vi "data_waypoint_ref.vi"() -> ()   [LabVIEW 2019] (continued)
"Y"=530169.107673044}, {"X"=175301.515584441, "Y"=530169.1522306317}, {"X"=175301.5505684368, "Y"=530169.1965216612}, {"X"=175301.58586430468, "Y"=530169.2408384063}, {"X"=175301.621437572, "Y"=530169.2849046132}, {"X"=175301.65624651004, "Y"=530169.3287078214}, {"X"=175301.69067446323, "Y"=530169.3715787638}, {"X"=175301.72433513994, "Y"=530169.4131889531}, {"X"=175301.7572057744, "Y"=530169.4545273413}, {"X"=175301.7897156011, "Y"=530169.4957669071}, {"X"=175301.82262842666, "Y"=530169.5363948606}, {"X"=175301.85541520052, "Y"=530169.5775315022}, {"X"=175301.88877971005, "Y"=530169.6193356836}, {"X"=175301.92198627733, "Y"=530169.6622479695}, {"X"=175301.9549979493, "Y"=530169.7066524813}, {"X"=175301.98874946675, "Y"=530169.7514277223}, {"X"=175302.02408231725, "Y"=530169.7962715428}, {"X"=175302.05988879167, "Y"=530169.84162117}, {"X"=175302.09521931363, "Y"=530169.886875645}, {"X"=175302.12915909418, "Y"=530169.9324128029}, {"X"=175302.16313239714, "Y"=530169.9770042623}, {"X"=175302.19741865405, "Y"=530170.0198878336}, {"X"=175302.23161996814, "Y"=530170.0622022983}, {"X"=175302.2647214002, "Y"=530170.1043091388}, {"X"=175302.29732747353, "Y"=530170.1466471837}, {"X"=175302.32942471874, "Y"=530170.1900533064}, {"X"=175302.36214685687, "Y"=530170.2339004164}, {"X"=175302.39546431036, "Y"=530170.2777679664}, {"X"=175302.42970125427, "Y"=530170.3213508952}, {"X"=175302.46371953157, "Y"=530170.3649755353}, {"X"=175302.4970483943, "Y"=530170.409108309}, {"X"=175302.53014454423, "Y"=530170.452725684}, {"X"=175302.56359763598, "Y"=530170.4957338027}, {"X"=175302.59699459223, "Y"=530170.5389285439}, {"X"=175302.63076028306, "Y"=530170.5819079936}, {"X"=175302.6641188947, "Y"=530170.625916373}, {"X"=175302.6977430426, "Y"=530170.6704567027}, {"X"=175302.7314268824, "Y"=530170.7154141635}, {"X"=175302.76559054904, "Y"=530170.7605799701}, {"X"=175302.80000400502, "Y"=530170.8048449432}, {"X"=175302.83450216462, "Y"=530170.8486979064}, {"X"=175302.868423361, "Y"=530170.8930431358}, {"X"=175302.9020594507, "Y"=530170.9368298354}, {"X"=175302.93501567593, "Y"=530170.9804587241}, {"X"=175302.96820232505, "Y"=530171.0238283353}, {"X"=175303.0014239085, "Y"=530171.0667294834}, {"X"=175303.03441731303, "Y"=530171.1100519415}, {"X"=175303.06691230068, "Y"=530171.153469102}, {"X"=175303.09917383848, "Y"=530171.1964219182}, {"X"=175303.13118923537, "Y"=530171.2397117508}, {"X"=175303.1637000194, "Y"=530171.2824795955}, {"X"=175303.19595648517, "Y"=530171.3261138815}, {"X"=175303.22875163666, "Y"=530171.3703914051}, {"X"=175303.26162110508, "Y"=530171.4149395159}, {"X"=175303.2943639709, "Y"=530171.4604080732}, {"X"=175303.3270933593, "Y"=530171.5061119605}, {"X"=175303.36078521397, "Y"=530171.5507863855}, {"X"=175303.39476642053, "Y"=530171.5950592977}, {"X"=175303.42826067653, "Y"=530171.6391105651}, {"X"=175303.46060070378, "Y"=530171.683447147}, {"X"=175303.4932010295, "Y"=530171.7277418941}, {"X"=175303.5264554045, "Y"=530171.7715508118}, {"X"=175303.56027406864, "Y"=530171.815673263}, {"X"=175303.59372100336, "Y"=530171.8604982444}, {"X"=175303.62725594908, "Y"=530171.9051320691}, {"X"=175303.66013932397, "Y"=530171.9501906737}, {"X"=175303.69312924595, "Y"=530171.9947339906}, {"X"=175303.72571887134, "Y"=530172.0390054631}, {"X"=175303.75856571438, "Y"=530172.0833916041}, {"X"=175303.7914979888, "Y"=530172.1276121215}, {"X"=175303.82426099747, "Y"=530172.1724058269}, {"X"=175303.85658823774, "Y"=530172.2175126894}, {"X"=175303.8893403862, "Y"=530172.2622276273}, {"X"=175303.9219982045, "Y"=530172.3070960032}, {"X"=175303.95487855875, "Y"=530172.3514321018}, {"X"=175303.98756941865, "Y"=530172.395190523}, {"X"=175304.0198873744, "Y"=530172.4383540505}, {"X"=175304.05146210626, "Y"=530172.4803022576}, {"X"=175304.08243248635, "Y"=530172.5218682386}, {"X"=175304.11302771606, "Y"=530172.5638781629}, {"X"=175304.14440576072, "Y"=530172.6058125234}, {"X"=175304.17647083785, "Y"=530172.6485317448}, {"X"=175304.2092485257, "Y"=530172.6916983553}, {"X"=175304.2421544904, "Y"=530172.7351098659}, {"X"=175304.27474581596, "Y"=530172.7793591394}, {"X"=175304.30713692037, "Y"=530172.8241972291}, {"X"=175304.33966600779, "Y"=530172.8692668731}, {"X"=175304.3725380399, "Y"=530172.9146862191}, {"X"=175304.40615073708, "Y"=530172.9595551069}, {"X"=175304.43922888403, "Y"=530173.0045820643}, {"X"=175304.47193721798, "Y"=530173.0500607167}, {"X"=175304.50408048517, "Y"=530173.095561017}, {"X"=175304.53664703757, "Y"=530173.1407204481}, {"X"=175304.57019344828, "Y"=530173.1850401526}, {"X"=175304.60417604624, "Y"=530173.229188761}, {"X"=175304.63733822326, "Y"=530173.274475177}, {"X"=175304.67012666404, "Y"=530173.3200845581}, {"X"=175304.70293440312, "Y"=530173.3656295104}, {"X"=175304.73601901694, "Y"=530173.4107485677}, {"X"=175304.7688052838, "Y"=530173.4550216836}, {"X"=175304.80180875398, "Y"=530173.4984595454}, {"X"=175304.83439683876, "Y"=530173.5410129662}, {"X"=175304.86641084577, "Y"=530173.5832384543}, {"X"=175304.89706473134, "Y"=530173.6259163404}, {"X"=175304.92851563115, "Y"=530173.6676274072}, {"X"=175304.96001501603, "Y"=530173.7089609802}, {"X"=175304.9911972434, "Y"=530173.7511778257}, {"X"=175305.0218017102, "Y"=530173.7939191228}, {"X"=175305.0528701443, "Y"=530173.8368965593}, {"X"=175305.0845467455, "Y"=530173.8803494384}, {"X"=175305.11676661787, "Y"=530173.9241980441}, {"X"=175305.1485606208, "Y"=530173.9687116023}, {"X"=175305.1810053819, "Y"=530174.0134252321}, {"X"=175305.21403351048, "Y"=530174.0580150564}, {"X"=175305.24728412752, "Y"=530174.1035575917}, {"X"=175305.28061614945, "Y"=530174.1499689076}, {"X"=175305.31471056672, "Y"=530174.1962902915}, {"X"=175305.3486507356, "Y"=530174.243170392}, {"X"=175305.3823800229, "Y"=530174.2900289173}, {"X"=175305.4154933949, "Y"=530174.3367893738}, {"X"=175305.4486278848, "Y"=530174.3826019497}, {"X"=175305.48151879795, "Y"=530174.4275195878}, {"X"=175305.5138967311, "Y"=530174.4724010066}, {"X"=175305.54595081756, "Y"=530174.517701799}, {"X"=175305.57926572644, "Y"=530174.562519407}, {"X"=175305.61313334163, "Y"=530174.6076283868}, {"X"=175305.64742550213, "Y"=530174.6531223445}, {"X"=175305.68094282097, "Y"=530174.6995930464}, {"X"=175305.7142195681, "Y"=530174.7464862061}, {"X"=175305.74732664338, "Y"=530174.7932144965}, {"X"=175305.78057287785, "Y"=530174.8402742251}, {"X"=175305.8133739154, "Y"=530174.8877536852}, {"X"=175305.84608374408, "Y"=530174.9352422942}, {"X"=175305.8802467283, "Y"=530174.9825878779}, {"X"=175305.91585264518, "Y"=530175.02962732}, {"X"=175305.95117603574, "Y"=530175.0772802396}, {"X"=175305.98675250847, "Y"=530175.1248480605}, {"X"=175306.0226269634, "Y"=530175.1719366532}, {"X"=175306.05766248834, "Y"=530175.219295199}, {"X"=175306.09146300732, "Y"=530175.2665819227}, {"X"=175306.1256061778, "Y"=530175.3138176922}, {"X"=175306.15987830423, "Y"=530175.3612284362}, {"X"=175306.19375731278, "Y"=530175.4089977182}, {"X"=175306.2272617157, "Y"=530175.4570955143}, {"X"=175306.26149442443, "Y"=530175.5043554353}, {"X"=175306.29601557076, "Y"=530175.5512049651}, {"X"=175306.33110052024, "Y"=530175.5979052205}, {"X"=175306.3664420601, "Y"=530175.6445070498}, {"X"=175306.40137430347, "Y"=530175.6922876495}, {"X"=175306.43611313298, "Y"=530175.7405627077}, {"X"=175306.47135692826, "Y"=530175.7888606924}, {"X"=175306.50683563814, "Y"=530175.836619701}, {"X"=175306.5427093849, "Y"=530175.8837704501}, {"X"=175306.57804036967, "Y"=530175.9312979346}, {"X"=175306.61314321528, "Y"=530175.9786596134}, {"X"=175306.64723720393, "Y"=530176.0260398111}, {"X"=175306.68197792507, "Y"=530176.0728576195}, {"X"=175306.71729545467, "Y"=530176.1191287831}, {"X"=175306.75288187485, "Y"=530176.1655689615}, {"X"=175306.78805515857, "Y"=530176.2121868278}, {"X"=175306.82317604765, "Y"=530176.2593597791}, {"X"=175306.85816065417, "Y"=530176.3068771907}, {"X"=175306.89302999235, "Y"=530176.3543549852}, {"X"=175306.92829042548, "Y"=530176.4019892259}, {"X"=175306.96434128538, "Y"=530176.4494269079}, {"X"=175307.0002629, "Y"=530176.4974909314}, {"X"=175307.03651319438, "Y"=530176.5461732863}, {"X"=175307.07280654478, "Y"=530176.5944370972}, {"X"=175307.10929617652, "Y"=530176.6425793526}, {"X"=175307.1459389947, "Y"=530176.6904026284}, {"X"=175307.1830941412, "Y"=530176.738340926}, {"X"=175307.2198662148, "Y"=530176.7870406077}, {"X"=175307.25608431565, "Y"=530176.836519937}, {"X"=175307.2923623031, "Y"=530176.8870823126}, {"X"=175307.32952882035, "Y"=530176.9370727075}, {"X"=175307.36630468437, "Y"=530176.9870564856}, {"X"=175307.40306440124, "Y"=530177.0369715019}, {"X"=175307.43982546963, "Y"=530177.0867444496}, {"X"=175307.47700678377, "Y"=530177.1363463515}, {"X"=175307.51413816065, "Y"=530177.1855366402}, {"X"=175307.55166098283, "Y"=530177.2347013578}, {"X"=175307.58907466935, "Y"=530177.2841050166}, {"X"=175307.62627763985, "Y"=530177.3341430286}, {"X"=175307.66311196302, "Y"=530177.3850267321}, {"X"=175307.7005225817, "Y"=530177.4357899772}, {"X"=175307.73824461747, "Y"=530177.486425782}, {"X"=175307.77605915256, "Y"=530177.5362899586}, {"X"=175307.81286147056, "Y"=530177.5865344778}, {"X"=175307.84951953805, "Y"=530177.6365241562}, {"X"=175307.88651088442, "Y"=530177.6859901074}, {"X"=175307.92401568915, "Y"=530177.7353546531}, {"X"=175307.9616221725, "Y"=530177.7846556385}, {"X"=175307.99953877402, "Y"=530177.8345883267}, {"X"=175308.03749193915, "Y"=530177.884904919}, {"X"=175308.07523145544, "Y"=530177.9354618721}, {"X"=175308.11299889255, "Y"=530177.9858755714}, {"X"=175308.15146935455, "Y"=530178.0352905402}, {"X"=175308.1892898605, "Y"=530178.0844787983}, {"X"=175308.2265397046, "Y"=530178.1335943816}, {"X"=175308.26328121778, "Y"=530178.1833474154}, {"X"=175308.30082930517, "Y"=530178.2326729915}, {"X"=175308.3391933072, "Y"=530178.2817331203}, {"X"=175308.37776592822, "Y"=530178.3309480151}, {"X"=175308.41586902775, "Y"=530178.3798457655}, {"X"=175308.45360439137, "Y"=530178.4289987606}, {"X"=175308.49054393347, "Y"=530178.4786213585}, {"X"=175308.52805617274, "Y"=530178.5275064252}, {"X"=175308.56581533956, "Y"=530178.5760211812}, {"X"=175308.60384613005, "Y"=530178.6241300373}, {"X"=175308.6412520306, "Y"=530178.6727002201}, {"X"=175308.67826697233, "Y"=530178.7214602334}, {"X"=175308.71486306612, "Y"=530178.7711648659}, {"X"=175308.75246034496, "Y"=530178.8215513228}, {"X"=175308.7912765256, "Y"=530178.872557922}, {"X"=175308.83084101314, "Y"=530178.9247021361}, {"X"=175308.8709113982, "Y"=530178.9771833654}, {"X"=175308.9109508622, "Y"=530179.0296935422}, {"X"=175308.95094127575, "Y"=530179.0814902235}, {"X"=175308.99123117467, "Y"=530179.1321184501}, {"X"=175309.03012990014, "Y"=530179.1819827599}, {"X"=175309.0674750189, "Y"=530179.2309682134}, {"X"=175309.1034754659, "Y"=530179.2796402158}, {"X"=175309.13934451604, "Y"=530179.327610065}, {"X"=175309.1753644265, "Y"=530179.3756738087}, {"X"=175309.21217135477, "Y"=530179.4232857344}, {"X"=175309.24893715564, "Y"=530179.4707690383}, {"X"=175309.28518585657, "Y"=530179.5189197841}, {"X"=175309.32090653412, "Y"=530179.5670399042}, {"X"=175309.35713197305, "Y"=530179.6151130308}, {"X"=175309.3934266228, "Y"=530179.6635266797}, {"X"=175309.42987620586, "Y"=530179.712513667}, {"X"=175309.46639058788, "Y"=530179.7624460628}, {"X"=175309.50371548356, "Y"=530179.8120852838}, {"X"=175309.5409782049, "Y"=530179.8619666371}, {"X"=175309.5787927472, "Y"=530179.9121404743}, {"X"=175309.61645778242, "Y"=530179.9635788811}, {"X"=175309.65459812188, "Y"=530180.0163932223}, {"X"=175309.69325909083, "Y"=530180.0694357668}, {"X"=175309.7317165625, "Y"=530180.122557711}, {"X"=175309.76908308847, "Y"=530180.1751967588}, {"X"=175309.80636802042, "Y"=530180.2269015467}, {"X"=175309.84373904276, "Y"=530180.2774640337}, {"X"=175309.88096197287, "Y"=530180.3267706002}, {"X"=175309.91734318458, "Y"=530180.3757034084}, {"X"=175309.9532567708, "Y"=530180.4237596989}, {"X"=175309.98798831712, "Y"=530180.472282293}, {"X"=175310.02238339974, "Y"=530180.5208502738}, {"X"=175310.0573020126, "Y"=530180.5694289177}, {"X"=175310.09330661935, "Y"=530180.6183128951}, {"X"=175310.12955154193, "Y"=530180.6672871724}, {"X"=175310.1658978246, "Y"=530180.7169914382}, {"X"=175310.20254698073, "Y"=530180.7669722736}, {"X"=175310.23967130386, "Y"=530180.817684213}, {"X"=175310.2773086728, "Y"=530180.8690550049}, {"X"=175310.3148211599, "Y"=530180.9201309427}, {"X"=175310.3511979726, "Y"=530180.9723744758}, {"X"=175310.38740139623, "Y"=530181.0252955357}, {"X"=175310.42416107788, "Y"=530181.0797110443}, {"X"=175310.4624049127, "Y"=530181.1348802013}, {"X"=175310.50164816767, "Y"=530181.1901351993}, {"X"=175310.54203527907, "Y"=530181.244894042}, {"X"=175310.58194975206, "Y"=530181.2991792613}, {"X"=175310.62001042886, "Y"=530181.3529172424}, {"X"=175310.65622358862, "Y"=530181.4049370685}, {"X"=175310.69123930926, "Y"=530181.4558061787}, {"X"=175310.72519802517, "Y"=530181.5047872087}, {"X"=175310.75874079563, "Y"=530181.5520969089}, {"X"=175310.79136085967, "Y"=530181.5980020331}, {"X"=175310.82360926468, "Y"=530181.6437328964}, {"X"=175310.85623968006, "Y"=530181.6907456301}, {"X"=175310.8897590421, "Y"=530181.7388267526}, {"X"=175310.9243145624, "Y"=530181.7880357637}, {"X"=175310.959343698, "Y"=530181.8383487933}, {"X"=175310.99435753067, "Y"=530181.8885797397}, {"X"=175311.0290962056, "Y"=530181.9392199271}, {"X"=175311.06388729028, "Y"=530181.990211786}, {"X"=175311.09868500763, "Y"=530182.0416486778}, {"X"=175311.13335366588, "Y"=530182.0931758506}, {"X"=175311.16810784728, "Y"=530182.1445684781}, {"X"=175311.20274703568, "Y"=530182.1960147172}, {"X"=175311.2379057422, "Y"=530182.2467135971}, {"X"=175311.27227776014, "Y"=530182.2976745092}, {"X"=175311.30606672564, "Y"=530182.3482675583}, {"X"=175311.3395601565, "Y"=530182.3986683643}, {"X"=175311.37393442274, "Y"=530182.448891213}, {"X"=175311.40852775157, "Y"=530182.4980068854}, {"X"=175311.44232597886, "Y"=530182.5478374333}, {"X"=175311.475157056, "Y"=530182.5983112288}, {"X"=175311.50801931764, "Y"=530182.6491478536}, {"X"=175311.54183613407, "Y"=530182.6998740053}, {"X"=175311.57663097818, "Y"=530182.7503397807}, {"X"=175311.61155363472, "Y"=530182.8014932929}, {"X"=175311.64626777923, "Y"=530182.8537284222}, {"X"=175311.68068305723, "Y"=530182.906743557}, {"X"=175311.7154702105, "Y"=530182.9591049955}, {"X"=175311.75001092287, "Y"=530183.0102019231}, {"X"=175311.78433634012, "Y"=530183.0606824049}, {"X"=175311.8183494312, "Y"=530183.1100850247}, {"X"=175311.8516716377, "Y"=530183.1588970209}, {"X"=175311.88408727964, "Y"=530183.2072721894}, {"X"=175311.91671428684, "Y"=530183.2552338662}, {"X"=175311.94992222873, "Y"=530183.3031472128}, {"X"=175311.98340970423, "Y"=530183.3515336459}, {"X"=175312.01677082642, "Y"=530183.4009259832}, {"X"=175312.0510007853, "Y"=530183.4505787942}, {"X"=175312.08557931965, "Y"=530183.5009863878}, {"X"=175312.12013653468, "Y"=530183.5522741646}, {"X"=175312.1542311072, "Y"=530183.6031737451}, {"X"=175312.1881540991, "Y"=530183.6538618514}, {"X"=175312.22243575216, "Y"=530183.7045222601}, {"X"=175312.25757506452, "Y"=530183.7549559459}, {"X"=175312.29278177244, "Y"=530183.8060153938}, {"X"=175312.32824544844, "Y"=530183.8574059312}, {"X"=175312.36394127307, "Y"=530183.9094206324}, {"X"=175312.4001556887, "Y"=530183.9609732128}, {"X"=175312.43641827087, "Y"=530184.0123380839}, {"X"=175312.4721263033, "Y"=530184.0636879449}, {"X"=175312.5069555313, "Y"=530184.1153023272}, {"X"=175312.54130807726, "Y"=530184.1674741576}, {"X"=175312.57628509818, "Y"=530184.2193444809}, {"X"=175312.61243834853, "Y"=530184.2708817059}, {"X"=175312.64919719583, "Y"=530184.3226235745}, {"X"=175312.68595615213, "Y"=530184.375303274}, {"X"=175312.72274589876, "Y"=530184.4288108387}, {"X"=175312.76002624852, "Y"=530184.4819762268}, {"X"=175312.79754509203, "Y"=530184.5349156114}, {"X"=175312.83499864914, "Y"=530184.5870438805}, {"X"=175312.8714617927, "Y"=530184.639437001}, {"X"=175312.90760069605, "Y"=530184.6915169893}, {"X"=175312.94404201457, "Y"=530184.7425184103}, {"X"=175312.98059682967, "Y"=530184.792660466}, {"X"=175313.01660241385, "Y"=530184.8418874011}, {"X"=175313.0520811022, "Y"=530184.891164725}, {"X"=175313.08734580636, "Y"=530184.9402695426}, {"X"=175313.12239439436, "Y"=530184.9893805474}, {"X"=175313.15734865, "Y"=530185.0386427735}, {"X"=175313.19286568387, "Y"=530185.0874072288}, {"X"=175313.22880935456, "Y"=530185.1363668718}, {"X"=175313.2649331918, "Y"=530185.1854447369}, {"X"=175313.30088473303, "Y"=530185.2346696118}, {"X"=175313.33722131583, "Y"=530185.2841008937}, {"X"=175313.37432573305, "Y"=530185.3331847425}, {"X"=175313.41198690207, "Y"=530185.3824289885}, {"X"=175313.449257545, "Y"=530185.4320095631}, {"X"=175313.48641791966, "Y"=530185.4820455073}, {"X"=175313.52345464373, "Y"=530185.5322027901}, {"X"=175313.56054014363, "Y"=530185.581779473}, {"X"=175313.59761448327, "Y"=530185.6311763932}, {"X"=175313.63479581906, "Y"=530185.6799115203}, {"X"=175313.67125340502, "Y"=530185.7286254782}, {"X"=175313.7071050316, "Y"=530185.7767130446}, {"X"=175313.74212418348, "Y"=530185.8236565841}, {"X"=175313.77722887165, "Y"=530185.8701692459}, {"X"=175313.8128344303, "Y"=530185.915917957}, {"X"=175313.8479152154, "Y"=530185.9618358053}, {"X"=175313.8821893614, "Y"=530186.0081600237}, {"X"=175313.9155590152, "Y"=530186.0544491778}, {"X"=175313.94968215242, "Y"=530186.1009303334}, {"X"=175313.98505024164, "Y"=530186.1469527704}, {"X"=175314.021090573, "Y"=530186.1929521351}, {"X"=175314.0570167525, "Y"=530186.2398907787}, {"X"=175314.0929765313, "Y"=530186.2871078982}, {"X"=175314.12863386451, "Y"=530186.3353935948}, {"X"=175314.16455866926, "Y"=530186.3845663889}, {"X"=175314.20138941368, "Y"=530186.4342648024}, {"X"=175314.2386463122, "Y"=530186.4848942381}, {"X"=175314.2759694681, "Y"=530186.5360639819}, {"X"=175314.31256280615, "Y"=530186.5878574002}, {"X"=175314.34945666775, "Y"=530186.638833074}, {"X"=175314.3865433375, "Y"=530186.6888093075}, {"X"=175314.42391436658, "Y"=530186.7372930504}, {"X"=175314.46051972595, "Y"=530186.7847590921}, {"X"=175314.49610486344, "Y"=530186.8319939679}, {"X"=175314.53065131142, "Y"=530186.8787435716}, {"X"=175314.56469552708, "Y"=530186.925797649}, {"X"=175314.5991626018, "Y"=530186.9729659047}, {"X"=175314.63475583828, "Y"=530187.0199443783}, {"X"=175314.6702479863, "Y"=530187.0677866219}, {"X"=175314.70570368378, "Y"=530187.1158842411}, {"X"=175314.74113296997, "Y"=530187.1637366577}, {"X"=175314.7767761707, "Y"=530187.2114375022}, {"X"=175314.8127982049, "Y"=530187.2590428923}, {"X"=175314.84901318164, "Y"=530187.3068952105}, {"X"=175314.88495516544, "Y"=530187.354989174}, {"X"=175314.92082059308, "Y"=530187.4035550535}, {"X"=175314.9563999271, "Y"=530187.4521262179}, {"X"=175314.99203503237, "Y"=530187.5000867952}, {"X"=175315.027573906, "Y"=530187.5481553137}, {"X"=175315.06366672198, "Y"=530187.5957349675}, {"X"=175315.09989612902, "Y"=530187.6433741514}, {"X"=175315.13577743215, "Y"=530187.6919177884}, {"X"=175315.17143027333, "Y"=530187.7407861799}, {"X"=175315.2078786093, "Y"=530187.7896733094}, {"X"=175315.24473079812, "Y"=530187.8379388351}, {"X"=175315.28113080456, "Y"=530187.8863588558}, {"X"=175315.3168192751, "Y"=530187.9346944091}, {"X"=175315.35221031535, "Y"=530187.9824947795}, {"X"=175315.3872724083, "Y"=530188.0301884642}, {"X"=175315.4232301929, "Y"=530188.0770360122}, {"X"=175315.45946732393, "Y"=530188.1242933825}, {"X"=175315.49556506728, "Y"=530188.172942929}, {"X"=175315.53165468454, "Y"=530188.2221396589}, {"X"=175315.5681028295, "Y"=530188.2712643011}, {"X"=175315.6050792257, "Y"=530188.319897936}, {"X"=175315.64205526988, "Y"=530188.3684117062}, {"X"=175315.67818000304, "Y"=530188.4163031384}, {"X"=175315.71349551325, "Y"=530188.4634256088}, {"X"=175315.7479487243, "Y"=530188.5107026764}, {"X"=175315.78355792633, "Y"=530188.5570928828}, {"X"=175315.8199135922, "Y"=530188.6030968745}, {"X"=175315.85587449878, "Y"=530188.6498034624}, {"X"=175315.890835794, "Y"=530188.6969602753}, {"X"=175315.92577562438, "Y"=530188.7449473259}, {"X"=175315.96154261148, "Y"=530188.7925767798}, {"X"=175315.99833612668, "Y"=530188.8407736705}, {"X"=175316.03534774587, "Y"=530188.8896380548}, {"X"=175316.07250852248, "Y"=530188.9386196402}, {"X"=175316.10918241073, "Y"=530188.9883018779}, {"X"=175316.14599503172, "Y"=530189.0375697273}, {"X"=175316.18267309142, "Y"=530189.0859634053}, {"X"=175316.21865495804, "Y"=530189.1340705757}, {"X"=175316.2542279634, "Y"=530189.1823032569}, {"X"=175316.28991713698, "Y"=530189.2311815331}, {"X"=175316.32575928187, "Y"=530189.2802680123}, {"X"=175316.36204323257, "Y"=530189.3298859186}, {"X"=175316.39863125872, "Y"=530189.3786882918}, {"X"=175316.43458270805, "Y"=530189.426994219}, {"X"=175316.4692830125, "Y"=530189.4751606653}, {"X"=175316.5038935927, "Y"=530189.5220388316}, {"X"=175316.5382121839, "Y"=530189.5681254207}, {"X"=175316.57219325224, "Y"=530189.6144993486}, {"X"=175316.60615941638, "Y"=530189.6612262579}, {"X"=175316.64103085897, "Y"=530189.7085542566}, {"X"=175316.67637426974, "Y"=530189.7564302428}, {"X"=175316.71164391257, "Y"=530189.8054218558}, {"X"=175316.74676780688, "Y"=530189.8548511842}, {"X"=175316.78219569896, "Y"=530189.9043395466}, {"X"=175316.8177323982, "Y"=530189.9537787547}, {"X"=175316.85369295246, "Y"=530190.0021701136}, {"X"=175316.8896444052, "Y"=530190.050779032}, {"X"=175316.92564777914, "Y"=530190.1001735788}, {"X"=175316.9620438199, "Y"=530190.1499565273}, {"X"=175316.99894420846, "Y"=530190.1998534118}, {"X"=175317.03558734115, "Y"=530190.2499219743}, {"X"=175317.07208662984, "Y"=530190.3004748595}, {"X"=175317.1083717217, "Y"=530190.3504823267}, {"X"=175317.1443335403, "Y"=530190.400203296}, {"X"=175317.18068957215, "Y"=530190.4502371901}, {"X"=175317.21824675493, "Y"=530190.4999789775}, {"X"=175317.25626110364, "Y"=530190.5500545918}, {"X"=175317.29395553737, "Y"=530190.6003819788}, {"X"=175317.3309519411, "Y"=530190.6512985411}, {"X"=175317.36805747618, "Y"=530190.7025765971}, {"X"=175317.40498688072, "Y"=530190.7539028961}, {"X"=175317.4429407785, "Y"=530190.8048066457}, {"X"=175317.48180363432, "Y"=530190.8554568817}, {"X"=175317.52073454688, "Y"=530190.9072578424}, {"X"=175317.55972893158, "Y"=530190.9592550602}, {"X"=175317.59894806604, "Y"=530191.0108720445}, {"X"=175317.6377611856, "Y"=530191.0620784669}, {"X"=175317.67635760055, "Y"=530191.1127916438}, {"X"=175317.7140501114, "Y"=530191.1633687577}, {"X"=175317.75095119307, "Y"=530191.2141035862}, {"X"=175317.78765461638, "Y"=530191.2650953768}, {"X"=175317.82558087553, "Y"=530191.3156396138}, {"X"=175317.86396142832, "Y"=530191.3661447766}, {"X"=175317.90213229894, "Y"=530191.4170345672}, {"X"=175317.94015622098, "Y"=530191.4673554361}, {"X"=175317.97785589864, "Y"=530191.5182610467}, {"X"=175318.0155045048, "Y"=530191.5692700257}, {"X"=175318.05364278206, "Y"=530191.620222066}, {"X"=175318.09153813362, "Y"=530191.6719994495}, {"X"=175318.1293183478, "Y"=530191.7246817079}, {"X"=175318.16774718426, "Y"=530191.7774419627}, {"X"=175318.20674981424, "Y"=530191.8298353782}, {"X"=175318.24521226567, "Y"=530191.8828796588}, {"X"=175318.28403795866, "Y"=530191.9350482963}, {"X"=175318.32304521388, "Y"=530191.9869078569}, {"X"=175318.36204793068, "Y"=530192.0384311461}, {"X"=175318.4005898055, "Y"=530192.0898758835}, {"X"=175318.43864458468, "Y"=530192.1416494689}, {"X"=175318.47640338843, "Y"=530192.1930820906}, {"X"=175318.51419378835, "Y"=530192.2441161796}, {"X"=175318.55208232062, "Y"=530192.2944862834}, {"X"=175318.58985834898, "Y"=530192.3451530531}, {"X"=175318.62736532633, "Y"=530192.3949971002}, {"X"=175318.66480275526, "Y"=530192.4440855398}, {"X"=175318.70216220792, "Y"=530192.4937657638}, {"X"=175318.74007465132, "Y"=530192.5435342542}, {"X"=175318.77838922056, "Y"=530192.5935956714}, {"X"=175318.81680214155, "Y"=530192.6436667865}, {"X"=175318.85473180335, "Y"=530192.6944685044}, {"X"=175318.893105015, "Y"=530192.7454908877}, {"X"=175318.93198027203, "Y"=530192.7964474163}, {"X"=175318.97074562093, "Y"=530192.847981396}, {"X"=175319.00950281188, "Y"=530192.8997518}, {"X"=175319.04856699263, "Y"=530192.9522948697}, {"X"=175319.08807038947, "Y"=530193.0047922492}, {"X"=175319.12802343152, "Y"=530193.0571762068}, {"X"=175319.16773230815, "Y"=530193.1099670911}, {"X"=175319.20749691897, "Y"=530193.1627333963}, {"X"=175319.24724586855, "Y"=530193.2155963047}, {"X"=175319.2868629425, "Y"=530193.2681954568}, {"X"=175319.32616219769, "Y"=530193.3205547077}, {"X"=175319.36573062692, "Y"=530193.3722783243}, {"X"=175319.4052265945, "Y"=530193.4237613154}, {"X"=175319.4445765745, "Y"=530193.4753002316}, {"X"=175319.48329824244, "Y"=530193.5267411147}, {"X"=175319.52202255937, "Y"=530193.5781808796}, {"X"=175319.56047417186, "Y"=530193.6296591858}, {"X"=175319.59880642896, "Y"=530193.6815151966}, {"X"=175319.6371569635, "Y"=530193.7326608438}, {"X"=175319.67575621096, "Y"=530193.7837424942}, {"X"=175319.71455607042, "Y"=530193.8343662901}, {"X"=175319.75346005248, "Y"=530193.8851551494}, {"X"=175319.7919885356, "Y"=530193.936569968}, {"X"=175319.83131689022, "Y"=530193.9879868631}, {"X"=175319.87087732382, "Y"=530194.0400046195}, {"X"=175319.91055584635, "Y"=530194.0927179083}, {"X"=175319.95018736875, "Y"=530194.1460129021}, {"X"=175319.99024830922, "Y"=530194.1992444766}, {"X"=175320.0305557881, "Y"=530194.2525741017}, {"X"=175320.0712095635, "Y"=530194.3052889514}, {"X"=175320.1119900287, "Y"=530194.3568103306}, {"X"=175320.15219124436, "Y"=530194.4083500657}, {"X"=175320.1921387411, "Y"=530194.458860601}, {"X"=175320.23155410215, "Y"=530194.5097467307}, {"X"=175320.2707313738, "Y"=530194.5609953767}, {"X"=175320.31042178915, "Y"=530194.6123379564}, {"X"=175320.35031262046, "Y"=530194.664057296}, {"X"=175320.3899530186, "Y"=530194.7158606148}, {"X"=175320.4297119804, "Y"=530194.767318418}, {"X"=175320.46997990887, "Y"=530194.8180544211}, {"X"=175320.51043847628, "Y"=530194.8688564525}, {"X"=175320.55115700723, "Y"=530194.9195034475}, {"X"=175320.5917810682, "Y"=530194.9702550462}, {"X"=175320.63193107033, "Y"=530195.0218526484}, {"X"=175320.67129892917, "Y"=530195.0737522215}, {"X"=175320.7100377912, "Y"=530195.1256225747}, {"X"=175320.74886255787, "Y"=530195.1768866911}, {"X"=175320.78829647583, "Y"=530195.2277594492}, {"X"=175320.82829674848, "Y"=530195.2781466381}, {"X"=175320.86779848064, "Y"=530195.3288871238}, {"X"=175320.90681250475, "Y"=530195.3794503614}, {"X"=175320.94602985482, "Y"=530195.429575715}, {"X"=175320.98480971038, "Y"=530195.4797301069}, {"X"=175321.02332181047, "Y"=530195.5292005048}, {"X"=175321.06128693797, "Y"=530195.57882124}, {"X"=175321.0995861466, "Y"=530195.6287894842}, {"X"=175321.1379527546, "Y"=530195.679084939}, {"X"=175321.17684378868, "Y"=530195.7290947222}, {"X"=175321.215752246, "Y"=530195.7787049029}, {"X"=175321.25457779068, "Y"=530195.8284340859}, {"X"=175321.2935347585, "Y"=530195.877373769}, {"X"=175321.33197582242, "Y"=530195.9267866664}, {"X"=175321.37019807613, "Y"=530195.9761924401}, {"X"=175321.40871088055, "Y"=530196.0256029064}, {"X"=175321.44677992928, "Y"=530196.0747216789}, {"X"=175321.48483888872, "Y"=530196.1231224035}, {"X"=175321.52257193413, "Y"=530196.1715429577}, {"X"=175321.56068217533, "Y"=530196.2202121164}, {"X"=175321.59924221472, "Y"=530196.2700208839}, {"X"=175321.63872254826, "Y"=530196.3210178126}, {"X"=175321.67865082875, "Y"=530196.3731266094}, {"X"=175321.71942213873, "Y"=530196.4266546473}, {"X"=175321.76037410757, "Y"=530196.4798691729}, {"X"=175321.80112038535, "Y"=530196.533019933}, {"X"=175321.8411714933, "Y"=530196.5856289156}, {"X"=175321.88069651256, "Y"=530196.6376612135}, {"X"=175321.9201304299, "Y"=530196.6885384173}, {"X"=175321.95949093453, "Y"=530196.7391528002}, {"X"=175321.99841810143, "Y"=530196.7900026427}, {"X"=175322.0373316636, "Y"=530196.8410456412}, {"X"=175322.0760458568, "Y"=530196.8926663568}, {"X"=175322.1152349461, "Y"=530196.9440259628}, {"X"=175322.1544901605, "Y"=530196.9952810451}, {"X"=175322.19440987587, "Y"=530197.0465907722}, {"X"=175322.23411659995, "Y"=530197.0980642746}, {"X"=175322.27372288413, "Y"=530197.1497212022}, {"X"=175322.31351665533, "Y"=530197.2012765786}, {"X"=175322.3533722951, "Y"=530197.2530859321}, {"X"=175322.39274468354, "Y"=530197.3041264676}, {"X"=175322.4312461575, "Y"=530197.3551040938}, {"X"=175322.4689193067, "Y"=530197.4054426665}, {"X"=175322.50720476272, "Y"=530197.454959244}, {"X"=175322.5459091693, "Y"=530197.5032659507}, {"X"=175322.58469188528, "Y"=530197.5513948477}, {"X"=175322.62243093, "Y"=530197.6003503415}, {"X"=175322.66002250477, "Y"=530197.64946276}, {"X"=175322.69777533837, "Y"=530197.6982894691}, {"X"=175322.7353187513, "Y"=530197.7469891632}, {"X"=175322.77224196383, "Y"=530197.7959381866}, {"X"=175322.80897855092, "Y"=530197.8452817602}, {"X"=175322.84632591892, "Y"=530197.8941851374}, {"X"=175322.88443607936, "Y"=530197.9437333102}, {"X"=175322.92386567718, "Y"=530197.9931510669}, {"X"=175322.96401642516, "Y"=530198.0432104138}, {"X"=175323.00403330493, "Y"=530198.0938306333}, {"X"=175323.04346028506, "Y"=530198.1450630171}, {"X"=175323.08229208103, "Y"=530198.196318245}, {"X"=175323.12123135975, "Y"=530198.2470748299}, {"X"=175323.15985042084, "Y"=530198.2982807423}, {"X"=175323.1988480503, "Y"=530198.3486997583}, {"X"=175323.23756583783, "Y"=530198.3991429065}, {"X"=175323.27665734818, "Y"=530198.4495583154}, {"X"=175323.31587152585, "Y"=530198.4992186585}, {"X"=175323.35479760286, "Y"=530198.5488043812}, {"X"=175323.39322686996, "Y"=530198.5981307524}, {"X"=175323.4315682364, "Y"=530198.6476860173}, {"X"=175323.46929583582, "Y"=530198.6969700654}, {"X"=175323.50722869192, "Y"=530198.7461702713}, {"X"=175323.5459397161, "Y"=530198.7946223526}, {"X"=175323.58439744834, "Y"=530198.8427899504}, {"X"=175323.62209566595, "Y"=530198.8917222602}, {"X"=175323.65877359055, "Y"=530198.9410005299}, {"X"=175323.69556244335, "Y"=530198.9900487311}, {"X"=175323.73411028614, "Y"=530199.0387354754}, {"X"=175323.77350876122, "Y"=530199.0881155926}, {"X"=175323.81290300708, "Y"=530199.1384646274}, {"X"=175323.85108638834, "Y"=530199.1891157913}, {"X"=175323.8888683214, "Y"=530199.2397037674}, {"X"=175323.92692682054, "Y"=530199.2885584359}, {"X"=175323.96485641086, "Y"=530199.3369540031}, {"X"=175324.00191990237, "Y"=530199.3851190561}, {"X"=175324.03842280654, "Y"=530199.4336209428}, {"X"=175324.07507156418, "Y"=530199.4829237162}, {"X"=175324.11335812218, "Y"=530199.5322183277}, {"X"=175324.15240360756, "Y"=530199.5817493182}, {"X"=175324.19127746008, "Y"=530199.6313518472}, {"X"=175324.2287002106, "Y"=530199.6817921636}, {"X"=175324.26553019526, "Y"=530199.7321742966}, {"X"=175324.30255214145, "Y"=530199.7815691971}, {"X"=175324.33997542586, "Y"=530199.8309895523}, {"X"=175324.3778948948, "Y"=530199.8801598336}, {"X"=175324.41578257747, "Y"=530199.929665387}, {"X"=175324.45303470409, "Y"=530199.9793193169}, {"X"=175324.49021220786, "Y"=530200.0288991062}, {"X"=175324.52719458667, "Y"=530200.0780943516}, {"X"=175324.56453317933, "Y"=530200.126432844}, {"X"=175324.6018519318, "Y"=530200.1752519632}, {"X"=175324.639619019, "Y"=530200.2247134796}, {"X"=175324.67763583743, "Y"=530200.2756559197}, {"X"=175324.71633669882, "Y"=530200.3275730183}, {"X"=175324.75549563722, "Y"=530200.3789316149}, {"X"=175324.79472103066, "Y"=530200.4299981245}, {"X"=175324.83290145468, "Y"=530200.4805516311}, {"X"=175324.8698345541, "Y"=530200.5307581061}, {"X"=175324.90571872293, "Y"=530200.5803106372}, {"X"=175324.94164630468, "Y"=530200.6292659377}, {"X"=175324.9781788097, "Y"=530200.6769974988}, {"X"=175325.01496359013, "Y"=530200.723770505}, {"X"=175325.05083836144, "Y"=530200.7713397482}, {"X"=175325.08665947133, "Y"=530200.8193353349}, {"X"=175325.12301564822, "Y"=530200.8679497532}, {"X"=175325.1597467984, "Y"=530200.9175597209}, {"X"=175325.1965801437, "Y"=530200.9678830262}, {"X"=175325.23368578497, "Y"=530201.0192288171}, {"X"=175325.27100025493, "Y"=530201.0708015133}, {"X"=175325.3086159226, "Y"=530201.1226851918}, {"X"=175325.3462306779, "Y"=530201.173658787}, {"X"=175325.38365508235, "Y"=530201.224064698}, {"X"=175325.42044835156, "Y"=530201.2740152087}, {"X"=175325.4568644001, "Y"=530201.3231078014}, {"X"=175325.49279309702, "Y"=530201.3721430111}, {"X"=175325.5287187662, "Y"=530201.4210528162}, {"X"=175325.56390410103, "Y"=530201.4709259429}, {"X"=175325.59903368057, "Y"=530201.5214163167}, {"X"=175325.63438651664, "Y"=530201.5719193501}, {"X"=175325.67106088204, "Y"=530201.6224007264}, {"X"=175325.70852292405, "Y"=530201.672954138}, {"X"=175325.74600077514, "Y"=530201.724963639}, {"X"=175325.78311414344, "Y"=530201.7780296917}, {"X"=175325.8204649508, "Y"=530201.8323125597}, {"X"=175325.85848104864, "Y"=530201.8872194239}, {"X"=175325.89734364732, "Y"=530201.9414190304}, {"X"=175325.93574889482, "Y"=530201.9949218861}, {"X"=175325.9731610076, "Y"=530202.0477684161}, {"X"=175326.00978406958, "Y"=530202.100076773}, {"X"=175326.0468937723, "Y"=530202.1507011494}, {"X"=175326.083703109, "Y"=530202.2006971186}, {"X"=175326.11978964065, "Y"=530202.2500903491}, {"X"=175326.15506203403, "Y"=530202.2991508055}, {"X"=175326.18999830802, "Y"=530202.3477727488}, {"X"=175326.2249742177, "Y"=530202.3954179}, {"X"=175326.26010835878, "Y"=530202.4426541552}, {"X"=175326.2947142973, "Y"=530202.4894968602}, {"X"=175326.32881687392, "Y"=530202.536559692}, {"X"=175326.36266935102, "Y"=530202.5844190321}, {"X"=175326.39759400964, "Y"=530202.6330077152}, {"X"=175326.43383685724, "Y"=530202.683445973}, {"X"=175326.47190138185, "Y"=530202.7349532002}, {"X"=175326.51121043155, "Y"=530202.7876609504}, {"X"=175326.55136520957, "Y"=530202.8415015922}, {"X"=175326.59171968058, "Y"=530202.8960752623}, {"X"=175326.6321905429, "Y"=530202.9510703352}, {"X"=175326.6722261586, "Y"=530203.0062542596}, {"X"=175326.71219305095, "Y"=530203.0615638003}, {"X"=175326.75209383233, "Y"=530203.116381868}, {"X"=175326.7917454435, "Y"=530203.1711107733}, {"X"=175326.83161576497, "Y"=530203.2246126398}, {"X"=175326.87189651153, "Y"=530203.2770178622}, {"X"=175326.91170643645, "Y"=530203.3286631126}, {"X"=175326.9508110747, "Y"=530203.3796411991}, {"X"=175326.98866926372, "Y"=530203.4302678084}, {"X"=175327.02652639092, "Y"=530203.4799343928}, {"X"=175327.06383915478, "Y"=530203.5291353314}, {"X"=175327.1012313738, "Y"=530203.5773460448}, {"X"=175327.13767728163, "Y"=530203.62515778}, {"X"=175327.1733785629, "Y"=530203.6724767144}, {"X"=175327.20888498292, "Y"=530203.7192002304}, {"X"=175327.24457231665, "Y"=530203.7662961268}, {"X"=175327.28073190898, "Y"=530203.8137380134}, {"X"=175327.31828937924, "Y"=530203.8621169378}, {"X"=175327.3568467017, "Y"=530203.9113286342}, {"X"=175327.39573231337, "Y"=530203.9613273641}, {"X"=175327.4348463128, "Y"=530204.0118770179}, {"X"=175327.4746820218, "Y"=530204.0623568422}, {"X"=175327.51439785375, "Y"=530204.1136372288}, {"X"=175327.55409277766, "Y"=530204.1650364326}, {"X"=175327.59377426372, "Y"=530204.2166853956}, {"X"=175327.63384299536, "Y"=530204.2683875972}, {"X"=175327.67389632692, "Y"=530204.3193728758}, {"X"=175327.71366109003, "Y"=530204.3698262745}, {"X"=175327.75270769326, "Y"=530204.419750169}, {"X"=175327.7914221135, "Y"=530204.4690701697}, {"X"=175327.82960123813, "Y"=530204.517694761}, {"X"=175327.86709288435, "Y"=530204.5662825343}, {"X"=175327.9041485433, "Y"=530204.6145086712}, {"X"=175327.94210074993, "Y"=530204.6615801282}, {"X"=175327.9798551974, "Y"=530204.7091738019}, {"X"=175328.0173480477, "Y"=530204.7569702436}, {"X"=175328.05459147744, "Y"=530204.8057918225}, {"X"=175328.09215344326, "Y"=530204.8553971305}, {"X"=175328.13028118102, "Y"=530204.9055201834}, {"X"=175328.16931487413, "Y"=530204.9561744055}, {"X"=175328.20865300385, "Y"=530205.0073360448}, {"X"=175328.24843108968, "Y"=530205.0590047016}, {"X"=175328.28835976106, "Y"=530205.110072481}, {"X"=175328.3279304532, "Y"=530205.1607994803}, {"X"=175328.36635310898, "Y"=530205.2115076702}, {"X"=175328.4048222024, "Y"=530205.2614421498}, {"X"=175328.44354148043, "Y"=530205.3115112955}, {"X"=175328.48294085654, "Y"=530205.3621167176}, {"X"=175328.52195241617, "Y"=530205.4139774231}, {"X"=175328.56165370328, "Y"=530205.4657362077}, {"X"=175328.60110805032, "Y"=530205.5175612008}, {"X"=175328.6405652865, "Y"=530205.568864554}, {"X"=175328.6796272788, "Y"=530205.619805039}, {"X"=175328.71811733616, "Y"=530205.670242225}, {"X"=175328.75615469483, "Y"=530205.7197573447}, {"X"=175328.79388382484, "Y"=530205.7689803721}, {"X"=175328.83173539452, "Y"=530205.8179721874}, {"X"=175328.86998914456, "Y"=530205.8666753601}, {"X"=175328.90845591988, "Y"=530205.9152258562}, {"X"=175328.94701416916, "Y"=530205.9638582114}, {"X"=175328.98495470296, "Y"=530206.0135811617}, {"X"=175329.02283770952, "Y"=530206.063320929}, {"X"=175329.061211757, "Y"=530206.1137684488}, {"X"=175329.1004535877, "Y"=530206.1644198417}, {"X"=175329.13965264565, "Y"=530206.215584116}, {"X"=175329.17943126732, "Y"=530206.2665369152}, {"X"=175329.21919262805, "Y"=530206.3173443769}, {"X"=175329.25909633044, "Y"=530206.3683600716}, {"X"=175329.29923168753, "Y"=530206.4189333583}, {"X"=175329.33950991664, "Y"=530206.4692942395}, {"X"=175329.37883474256, "Y"=530206.5198543807}, {"X"=175329.4174794207, "Y"=530206.5710624671}, {"X"=175329.45618161428, "Y"=530206.6222492951}, {"X"=175329.49601390955, "Y"=530206.6721808698}, {"X"=175329.53568236195, "Y"=530206.7218221434}, {"X"=175329.57487133163, "Y"=530206.7710708327}, {"X"=175329.61317725817, "Y"=530206.8203476531}, {"X"=175329.65166145592, "Y"=530206.868802654}, {"X"=175329.69034324563, "Y"=530206.9169784943}, {"X"=175329.72884437937, "Y"=530206.9657686227}, {"X"=175329.76712680032, "Y"=530207.0151864667}, {"X"=175329.80580621227, "Y"=530207.0652579557}, {"X"=175329.84515547164, "Y"=530207.1153951712}, {"X"=175329.88507176263, "Y"=530207.1655773262}, {"X"=175329.92491169384, "Y"=530207.2159972164}, {"X"=175329.96473889175, "Y"=530207.2666047115}, {"X"=175330.0045233484, "Y"=530207.3177372969}, {"X"=175330.04477562633, "Y"=530207.3689128957}, {"X"=175330.08507576596, "Y"=530207.4206987759}, {"X"=175330.12605519747, "Y"=530207.4715492621}, {"X"=175330.16637356245, "Y"=530207.5226070208}, {"X"=175330.20511206114, "Y"=530207.5740934082}, {"X"=175330.24271986936, "Y"=530207.6257351815}, {"X"=175330.2810642061, "Y"=530207.6763248568}, {"X"=175330.31986330473, "Y"=530207.7258344068}, {"X"=175330.35768402094, "Y"=530207.775783018}, {"X"=175330.39437893714, "Y"=530207.8254430583}, {"X"=175330.4313906394, "Y"=530207.874092192}, {"X"=175330.46888017948, "Y"=530207.921375898}, {"X"=175330.50616064473, "Y"=530207.9677490287}, {"X"=175330.5426012657, "Y"=530208.0146817855}, {"X"=175330.57887375378, "Y"=530208.0619724141}, {"X"=175330.61506270058, "Y"=530208.1103698179}, {"X"=175330.65235307286, "Y"=530208.1595009197}, {"X"=175330.6898371192, "Y"=530208.2097268798}, {"X"=175330.72784761153, "Y"=530208.2603519466}, {"X"=175330.7657841934, "Y"=530208.3108440499}, {"X"=175330.80350983172, "Y"=530208.361594262}, {"X"=175330.84116910724, "Y"=530208.4123679763}, {"X"=175330.8800341823, "Y"=530208.4632258139}, {"X"=175330.91904552278, "Y"=530208.5144217251}, {"X"=175330.95728834765, "Y"=530208.5660349927}, {"X"=175330.99433718255, "Y"=530208.6182655349}, {"X"=175331.0318488113, "Y"=530208.6688343638}, {"X"=175331.06905319763, "Y"=530208.7185461762}, {"X"=175331.10566655878, "Y"=530208.7675871584}, {"X"=175331.14137250715, "Y"=530208.8168039559}, {"X"=175331.17715414436, "Y"=530208.8661548237}, {"X"=175331.21332360696, "Y"=530208.9154568233}, {"X"=175331.25029619085, "Y"=530208.9649606678}, {"X"=175331.2873574178, "Y"=530209.0144875587}, {"X"=175331.32414960433, "Y"=530209.0643948126}, {"X"=175331.36084215975, "Y"=530209.114159192}, {"X"=175331.3975425129, "Y"=530209.1638647242}, {"X"=175331.43446336297, "Y"=530209.2144497242}, {"X"=175331.47308668031, "Y"=530209.2647300402}, {"X"=175331.51153533268, "Y"=530209.315855475}, {"X"=175331.54889317372, "Y"=530209.3674425003}, {"X"=175331.5855494454, 
